vi "addImage.vi"(8 "error in (no error)":errorcluster, 9 "number of images":i32=3, 10 "ImageData":T1, 11 "AbsorptionAnalyser in":refnum<class "AbsorptionAnalyser.lvclass">) -> (0 "error out":errorcluster, 3 "AbsorptionAnalyser out":refnum<class "AbsorptionAnalyser.lvclass">)   [LabVIEW 2011, in "Tools.lvlib" / "Imaging.lvlib" / "AbsorptionAnalyser.lvclass"]
uses:
  AbsorptionAnalyser.lvclass
  AbsorptionAnalyser.lvclass/AbsorptionAnalyser.ctl
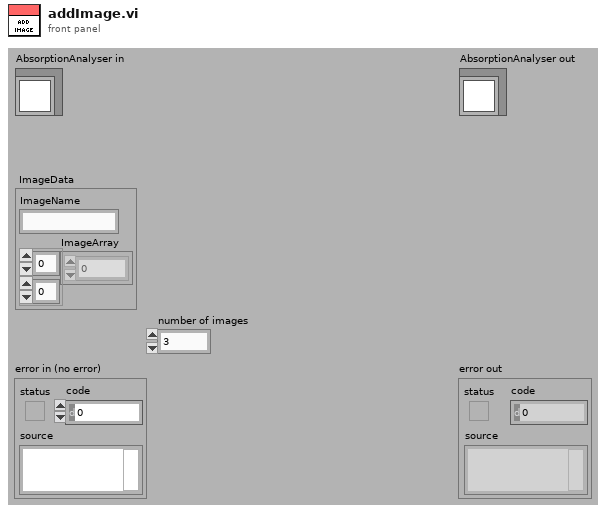
[diagram p1: front panel]
types:
  T1 = cluster{"ImageName":string, "ImageArray":sgl[][]}
  T2 = cluster{"ImageName":string, "ImageArray":sgl[][]}[]
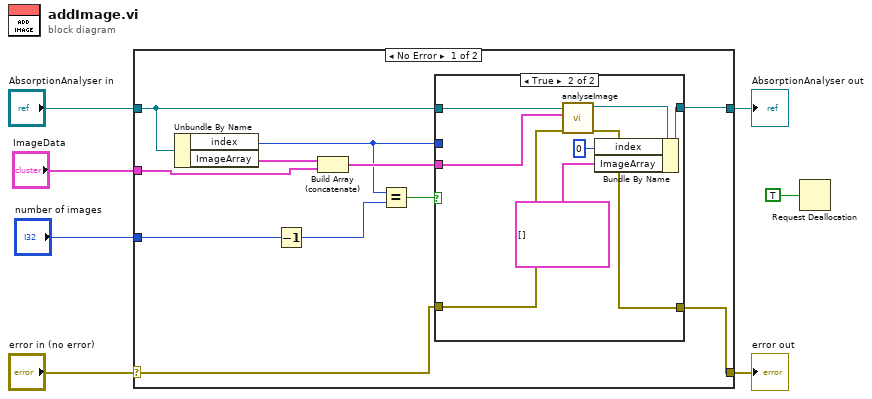
[diagram p0: block diagram]
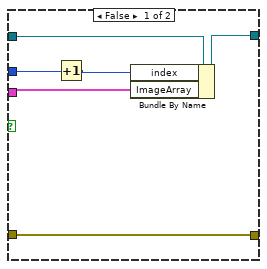
[diagram p2: hidden frame]
diagram:
  n1 = case shown="No Error" "error in (no error)" {
    selector: "error in (no error)" -> [w12 w34]
    tunnel: [w11 w34] -> w6
    tunnel: [w13 w33] -> w4
    tunnel: "AbsorptionAnalyser in" -> [w16 w33]
    tunnel: "ImageData" -> [w10 _]
    tunnel: "number of images" -> [w8 _]
    frame No Error {
      n2 = Unbundle By Name(w16) -> ("index"=w14:i32, "ImageArray"=w18:T2)
      n3 = Decrement(x=w8) -> (x-1=w9:i32)
      n4 = Build Array (concatenate)(w18, w10) -> (w15:T2)
      n5 = Equal?(x=w14, y=w9) -> (x = y?=w17:bool)
      n6 = case shown="True" w17 {
        tunnel: w16 -> [w23 w32]
        tunnel: w15 -> [w20 w29]
        tunnel: w14 -> [w24 _]
        tunnel: [w22 w27] -> w13
        tunnel: w12 -> [w19 w31]
        tunnel: [w19 w30] -> w11
        frame False {
          n7 = Increment(x=w24) -> (x+1=w21:i32)
          n8 = Bundle By Name(cluster=w23, "index"=w21, "ImageArray"=w20) -> (w22:refnum<class "AbsorptionAnalyser.lvclass">)
        }
        frame True {
          n9 = call-dynamic "analyseImage.vi"("error in (no error)"=w31, "Array"=w29, "AbsorptionAnalyser in"=w32) -> ("error out"=w30:errorcluster, "AbsorptionAnalyser out"=w28:refnum<class "AbsorptionAnalyser.lvclass">)  [unwired: 7 in]
          n10 = Bundle By Name(cluster=w28, "index"=0, "ImageArray"=T2 []) -> (w27:refnum<class "AbsorptionAnalyser.lvclass">)
        }
      }
    }
    frame Error {
    }
  }
  "error out" <- w6
  "AbsorptionAnalyser out" <- w4
  n11 = Request Deallocation(TRUE ("flag")) -> ()
